vi "applyTDWindow.vi"(1 "Sync Matrix Windows":bool, 2 "Retain Settings":bool, 3 "Sigma":dbl, 4 "Cursor 2 (ns)":dbl, 5 "Cursor 1 (ns)":dbl, 6 "Matrix":i32) -> ()   [LabVIEW 2012]
uses:
  bin/OVA32.dll
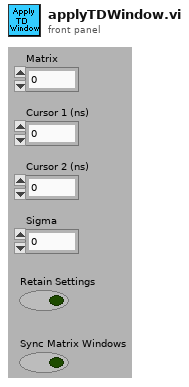
[diagram p1: front panel]
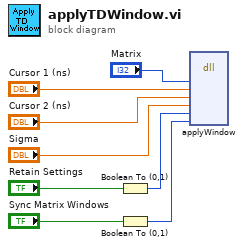
[diagram p0: block diagram]
diagram:
  n1 = Boolean To (0,1)(Boolean="Retain Settings") -> (0, 1=w2:i16)
  n2 = Boolean To (0,1)(Boolean="Sync Matrix Windows") -> (0, 1=w8:i16)
  n3 = dll-call lib="C:/_src/OVA5000_DSP_falcon/Software/LabVIEW/OVA/SDK/OVA_5000_SDK_v5.14.3/bin/OVA32.dll" fn="applyWindow"("matrix"="Matrix", "cursor1"="Cursor 1 (ns)", "curosor2"="Cursor 2 (ns)", "sigma"="Sigma", "save"=w2, "sync"=w8) -> ()  [unwired: 10 in, 2 out]
